vi "HAL Stage close.vi"   [LabVIEW 2016]
uses:
  new-h-nu-ixon/stage globals.vi
  C:/Program Files/Mad City Labs/NanoDrive/Labview 32-bit/Madlib.dll
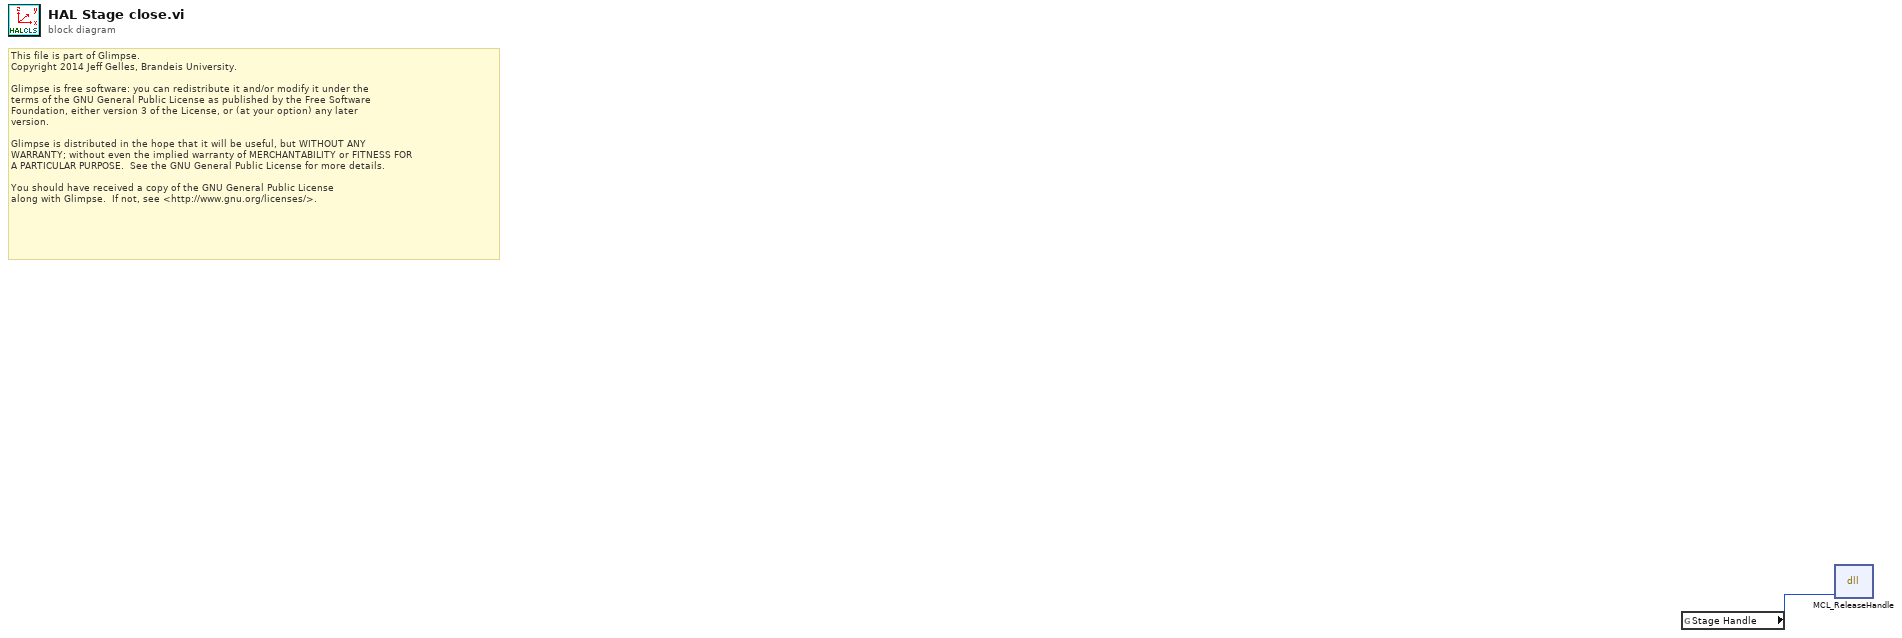
[diagram p0: block diagram]
diagram:
  # "This file is part of Glimpse. \nCopyright 2014 Jeff Gelles, Brandeis University.    \n\nGlimpse is free software: you can redistribute it and/or modify it under the \nterms of the GNU General Public License as published by the Free Software \nFoundation, either version 3 of the License, or (at your option) any later \nversion.\n\nGlimpse is distributed in the hope that it will be useful, but WITHOUT ANY \nWARRANTY; without even the implied warranty of MERCHANTABILITY or FITNESS FOR \nA PARTICULAR PURPOSE.  See the GNU General Public License for more details.\n\nYou should have received a copy of the GNU General Public License\nalong with Glimpse.  If not, see <http://www.gnu.org/licenses/>."
  n1 = global read "stage globals.vi" "Stage Handle"() -> (w1:i32)
  n2 = dll-call lib="C:/Program Files/Mad City Labs/NanoDrive/Labview 32-bit/MADLib.dll" fn="MCL_ReleaseHandle"("handle"=w1) -> ()  [unwired: 5 in, 2 out]
